vi "hamiltonian.vi"() -> ()   [LabVIEW 2024]
uses:
  <vilib>/Analysis/Matrix/Datatypes/ComplexMatrix.ctl
  <vilib>/Analysis/7linalg.llb/Real Eigenvalues and Vectors.vi
  <vilib>/Analysis/NI_AALPro.lvlib
  <vilib>/Analysis/Matrix/NI_Matrix.lvlib
panel:
  out "x^y 2":cdb
  out "x^y":cdb
  out "Probability distribution of superposition 2":cdb[](array[numeric])
  out "Array 2":dbl[](array[numeric])
  out "Array":dbl[](array[numeric])
  out "Potential":cluster{dbl[], dbl[]}(graph)
  out "Wave function of Superposition":cdb[](array[numeric])
  out "Probability distribution of superposition":cluster{i32[], dbl[]}(graph)
  out "factor first":cdb
  out "factor ground":cdb
  out "energy 1":cdb
  out "energy 0":cdb
  out "Probability Distribution First Excited State":cluster{i32[], "Eigenvectors":dbl[]}(graph)
  out "First Excited State":cluster{i32[], "Eigenvectors":dbl[]}(graph)
  out "Ground State":cluster{i32[], "Eigenvectors":dbl[]}(graph)
  out "Position":i32[](array[numeric])
  out "Ground State":cdb[](array[numeric])
  out "Eigenvectors":T1
  out "Eigenvalues":cdb[](array[numeric])
  out "Hamiltonian":dbl[][](array[numeric])
  in  "dimension size":i32
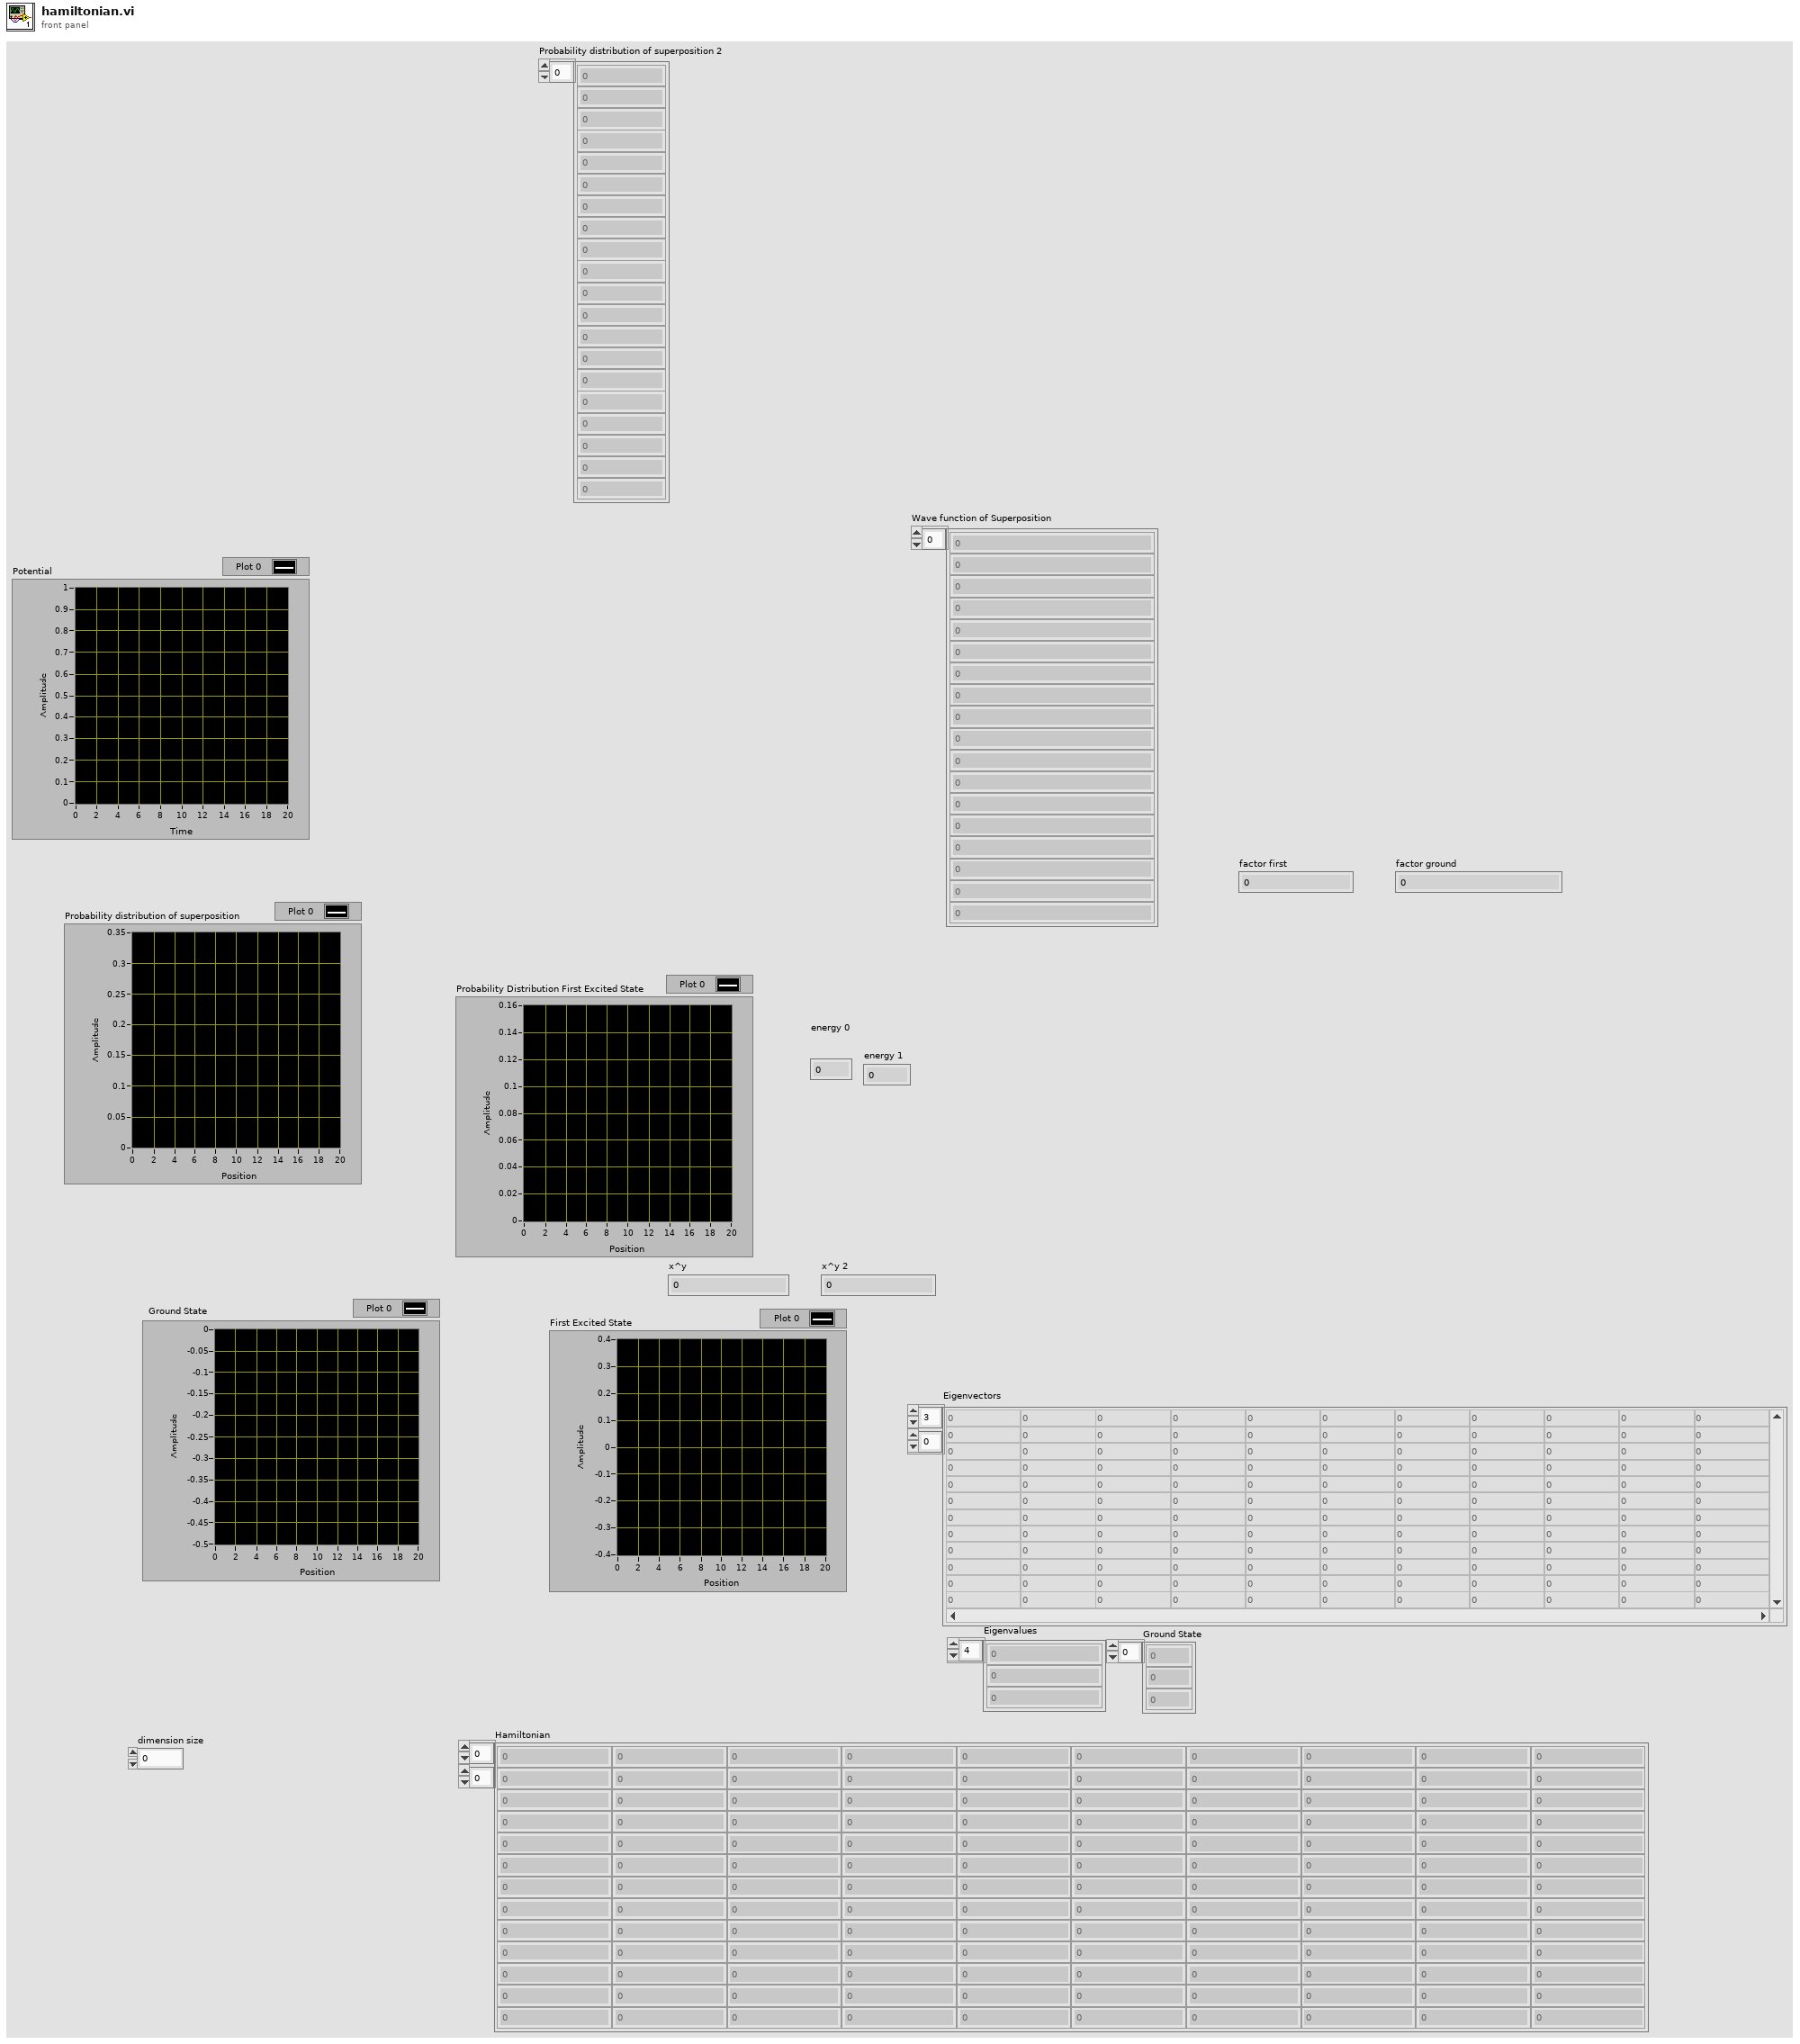
[diagram p1: front panel]
types:
  T1 = typedef "NI_Matrix.lvlib/ComplexMatrix.ctl" = cdb[][]
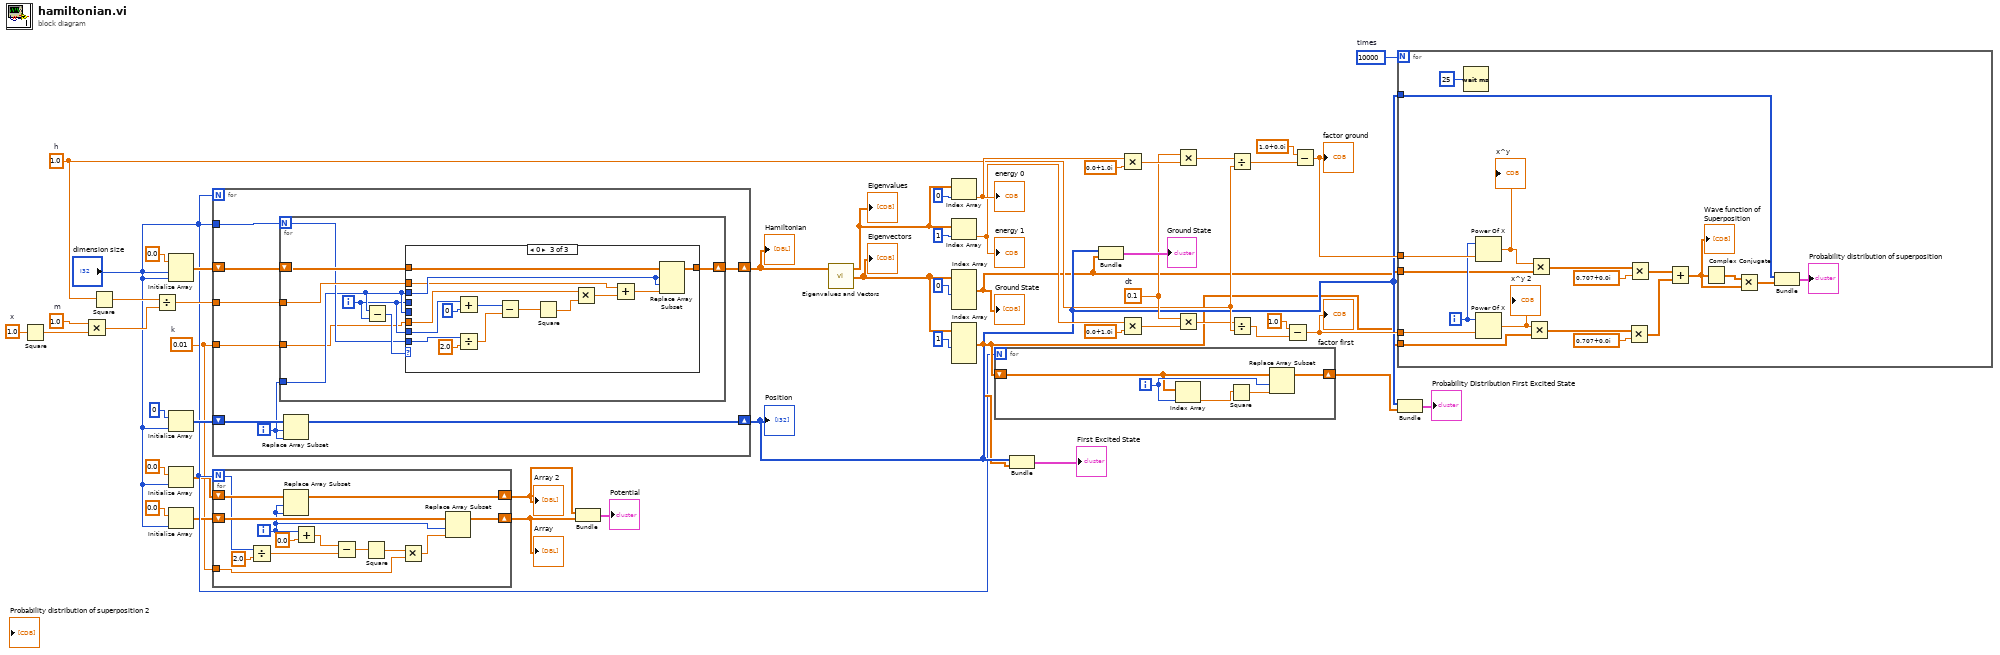
[diagram p0: block diagram]
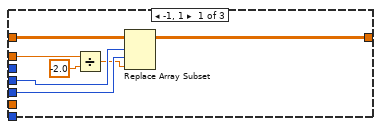
[diagram p2: hidden frame]
diagram:
  w23 = 10000  # times
  w18 = 0.1  # dt
  w5 = 0.01  # k
  w48 = 1.0  # x
  w47 = 1.0  # m
  w17 = 1.0  # h
  n1 = Square(x=w48) -> (x^2=w46:dbl)
  n2 = Multiply(x=w47, y=w46) -> (x*y=w44:dbl)
  n3 = Square(x=w17) -> (x^2=w45:dbl)
  n4 = Divide(x=w45, y=w44) -> (x/y=w43:dbl)
  n5 = Initialize Array(0.0 ("element"), "dimension size", "dimension size") -> (w49:dbl[][])
  n6 = Initialize Array(0 ("element"), "dimension size") -> (w39:i32[])
  n7 = Initialize Array(0.0 ("element"), "dimension size") -> (w7:dbl[])
  n8 = Initialize Array(0.0 ("element"), "dimension size") -> (w6:dbl[])
  n9 = for {
    N: "dimension size" -> [_]
    tunnel: "dimension size" -> [w58]
    shift-right: [w56] -> w42
    shift-left: w49 -> [w57]
    tunnel: w43 -> [w55]
    tunnel: w5 -> [w54]
    shift-right: [w52] -> w12
    shift-left: w39 -> [w53]
    i -> [w51]
    n10 = for {
      N: w58 -> [w62]
      tunnel: w51 -> [w61]
      shift-right: [w64] -> w56
      shift-left: w57 -> [w65]
      tunnel: w55 -> [w63]
      tunnel: w54 -> [w59]
      i -> [w60]
      n11 = Subtract(x=w61, y=w60) -> (x-y=w66:i32)
      n12 = case shown="0" w66 {
        tunnel: w65 -> [w73 w74 w89]
        tunnel: [w69 w74 w88] -> w64
        tunnel: w61 -> [_ _ w87]
        tunnel: w63 -> [w68 _ w86]
        tunnel: w62 -> [_ _ w83]
        tunnel: w60 -> [_ _ w82]
        tunnel: w61 -> [w72 _ _]
        tunnel: w60 -> [w71 _ _]
        tunnel: w59 -> [_ _ w76]
        frame -1, 1 {
          n13 = Divide(x=w68, y=-2.0) -> (x/y=w67:dbl)
          n14 = Replace Array Subset(array=w73, new element=w67, index (row)=w71, index (col)=w72) -> (w69:dbl[][])
        }
        frame 2, Default {
        }
        frame 0 {
          n15 = Add(x=w82, y=0) -> (x+y=w79:i32)
          n16 = Divide(x=w83, y=2.0) -> (x/y=w81:dbl)
          n17 = Subtract(x=w79, y=w81) -> (x-y=w85:dbl)
          n18 = Square(x=w85) -> (x^2=w77:dbl)
          n19 = Multiply(x=w76, y=w77) -> (x*y=w75:dbl)
          n20 = Add(x=w86, y=w75) -> (x+y=w80:dbl)
          n21 = Replace Array Subset(array=w89, new element=w80, index (row)=w87, index (col)=w87) -> (w88:dbl[][])
        }
      }
    }
    n22 = Replace Array Subset(array=w53, new element=w51, index=w51) -> (w52:i32[])
  }
  "Hamiltonian" <- w42
  "Position" <- w12
  n23 = for {
    N: "dimension size" -> [w97]
    tunnel: w5 -> [w94]
    shift-right: [w91] -> w4
    shift-left: w7 -> [w103]
    shift-right: [w92] -> w3
    shift-left: w6 -> [w102]
    i -> [w90]
    n24 = Divide(x=w97, y=2.0) -> (x/y=w99:dbl)
    n25 = Replace Array Subset(array=w103, new element=w90, index=w90) -> (w91:dbl[])
    n26 = Add(x=w90, y=0.0) -> (x+y=w100:dbl)
    n27 = Subtract(x=w100, y=w99) -> (x-y=w96:dbl)
    n28 = Square(x=w96) -> (x^2=w95:dbl)
    n29 = Multiply(x=w95, y=w94) -> (x*y=w93:dbl)
    n30 = Replace Array Subset(array=w102, new element=w93, index=w90) -> (w92:dbl[])
  }
  "Array" <- w3
  "Array 2" <- w4
  n31 = Bundle(w4, w3) -> (→"Potential":cluster{dbl[], dbl[]})  [unwired: 1 in]
  n32 = call-poly <vilib>:"Eigenvalues and Vectors.vi"("Input Matrix"=w42) -> ("Eigenvectors"=w37:T1, "Eigenvalues"=w32:cdb[])  [unwired: 2 in, 1 out]
  "Eigenvalues" <- w32
  "Eigenvectors" <- w37
  n33 = Index Array(array=w32, index=0) -> (element=w29:cdb)
  "energy 0" <- w29
  n34 = Index Array(array=w32, index=1) -> (element=w21:cdb)
  "energy 1" <- w21
  n35 = Index Array(array=w37, index (col) #1=0 ("disabled index (col)")) -> (element #1=w1:cdb[])  [unwired: 3 in, 1 out]
  "Ground State" <- w1
  n36 = Index Array(array=w37, index (col) #1=1 ("disabled index (col)")) -> (element #1=w11:cdb[])  [unwired: 3 in, 1 out]
  n37 = for {
    N: "dimension size" -> [_]
    shift-right: [w107] -> w34
    shift-left: w11 -> [w104]
    i -> [w105]
    n38 = Index Array(array=w104, index=w105) -> (element=w106:cdb)
    n39 = Square(x=w106) -> (x^2=w108:cdb)
    n40 = Replace Array Subset(array=w104, new element=w108, index=w105) -> (w107:cdb[])
  }
  n41 = Bundle(w12, "Eigenvectors"=w11) -> (→"First Excited State":cluster{i32[], "Eigenvectors":cdb[]})  [unwired: 1 in]
  n42 = Bundle(w12, "Eigenvectors"=w1) -> (→"Ground State":cluster{i32[], "Eigenvectors":cdb[]})  [unwired: 1 in]
  n43 = Multiply(x=w29, y=cdb 0.0+1.0i) -> (x*y=w27:cdb)
  n44 = Multiply(x=w21, y=cdb 0.0+1.0i) -> (x*y=w19:cdb)
  n45 = Multiply(x=w18, y=w27) -> (x*y=w26:cdb)
  n46 = Multiply(x=w18, y=w19) -> (x*y=w16:cdb)
  n47 = Divide(x=w26, y=w17) -> (x/y=w25:cdb)
  n48 = Divide(x=w16, y=w17) -> (x/y=w14:cdb)
  n49 = Subtract(x=1.0, y=w14) -> (x-y=w13:cdb)
  "factor first" <- w13
  n50 = Subtract(x=cdb 1.0+0.0i, y=w25) -> (x-y=w22:cdb)
  "factor ground" <- w22
  n51 = for {
    N: w23 -> [_]
    tunnel: w22 -> [w126]
    tunnel: w13 -> [w124]
    tunnel: w12 -> [w114]
    tunnel: w1 -> [w109]
    tunnel: w11 -> [w112]
    i -> [w125]
    n52 = Wait (ms)(milliseconds to wait=u32 25) -> ()  [unwired: 1 out]
    n53 = Power Of X(1:w126, 2:w125) -> (0:w127:cdb)
    "x^y" <- w127
    n54 = Power Of X(1:w124, 2:w125) -> (0:w123:cdb)
    "x^y 2" <- w123
    n55 = Multiply(x=w123, y=w112) -> (x*y=w121:cdb[])
    n56 = Multiply(x=w127, y=w109) -> (x*y=w110:cdb[])
    n57 = Multiply(x=w121, y=cdb 0.707+0.0i) -> (x*y=w118:cdb[])
    n58 = Multiply(x=w110, y=cdb 0.707+0.0i) -> (x*y=w119:cdb[])
    n59 = Add(x=w119, y=w118) -> (x+y=w116:cdb[])
    "Wave function of Superposition" <- w116
    n60 = Complex Conjugate(1:w116) -> (0:w117:cdb[])
    n61 = Multiply(x=w117, y=w116) -> (x*y=w115:cdb[])
    n62 = Bundle(w114, w115) -> (→"Probability distribution of superposition":cluster{i32[], cdb[]})  [unwired: 1 in]
  }
  n63 = Bundle(w12, "Eigenvectors"=w34) -> (→"Probability Distribution First Excited State":cluster{i32[], "Eigenvectors":cdb[]})  [unwired: 1 in]
